vi "Config - Load.vi"(8 "error in (no error)":errorcluster, 11 "Default Configuration":T1) -> (0 "error out":errorcluster, 3 "Configuration":T1)   [LabVIEW 2017]
doc: "Loads the configuration from the XML file. If file not found, uses the provided defaults."
uses:
  Controls/Configuration Data.ctl
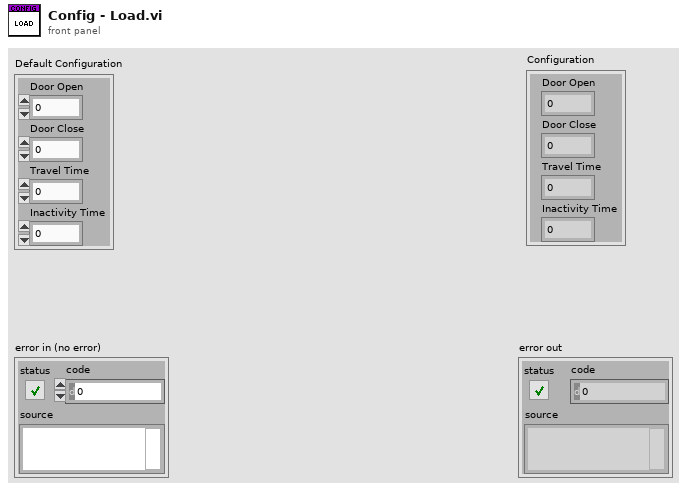
[diagram p1: front panel]
types:
  T1 = typedef "Configuration Data.ctl" = cluster{"Door Open":dbl, "Door Close":dbl, "Travel Time":dbl, "Inactivity Time":dbl}
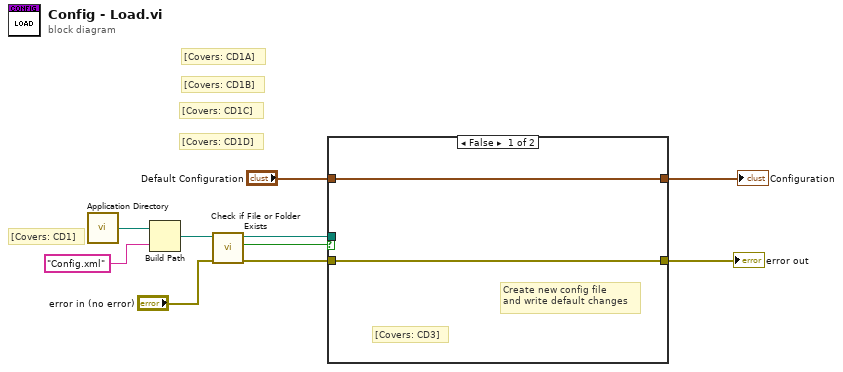
[diagram p0: block diagram]
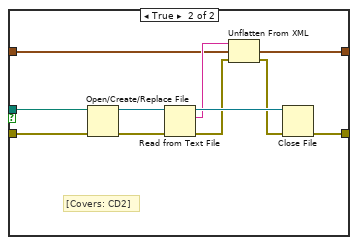
[diagram p2: hidden frame]
diagram:
  # "[Covers: CD1]"
  # "[Covers: CD1D]"
  # "[Covers: CD1C]"
  # "[Covers: CD1B]"
  # "[Covers: CD1A]"
  n1 = call <vilib>:"Application Directory.vi"() -> ("Application Directory"=w10:path)
  n2 = Build Path(base path=w10, name or relative path="Config.xml") -> (appended path=w8:path)
  n3 = call <vilib>:"Check if File or Folder Exists.vi"("error in (no error)"="error in (no error)", "path"=w8) -> ("error out"=w6:errorcluster, "file or folder exists?"=w7:bool, "dup path"=w5:path)  [unwired: 7 in]
  n4 = case shown="False" w7 {
    tunnel: w6 -> [w11 w23]
    tunnel: w5 -> [_ w22]
    tunnel: "Default Configuration" -> [w12 w15]
    tunnel: [w12 w14] -> w2
    tunnel: [w11 w13] -> w1
    frame False {
      # "Create new config file\nand write default changes"
      # "[Covers: CD3]"
    }
    frame True {
      # "[Covers: CD2]"
      n5 = Open/Create/Replace File(file path (use dialog)=w22, error in=w23) -> (refnum out=w20:refnum<file>, error out=w21:errorcluster)  [unwired: 4 in, 1 out]
      n6 = Read from Text File(file (use dialog)=w20, error in=w21) -> (refnum out=w19:refnum<file>, text=w16:string, error out=w18:errorcluster)  [unwired: 2 in, 1 out]
      n7 = Unflatten From XML(xml string=w16, type=w15, error in (no error)=w18) -> (value=w14:T1, error out=w17:errorcluster)
      n8 = Close File(refnum=w19, error in=w17) -> (error out=w13:errorcluster)  [unwired: 1 out]
    }
  }
  "error out" <- w1
  "Configuration" <- w2
